vi "Open.vi"(8 "error in (no error)":errorcluster, 11 "reference in":refnum<class "GarageDoor.lvclass">) -> (0 "error out":errorcluster, 3 "reference out":refnum<class "GarageDoor.lvclass">)   [LabVIEW 2020, in "GarageDoor.lvclass"]
uses:
  GarageDoor.lvclass
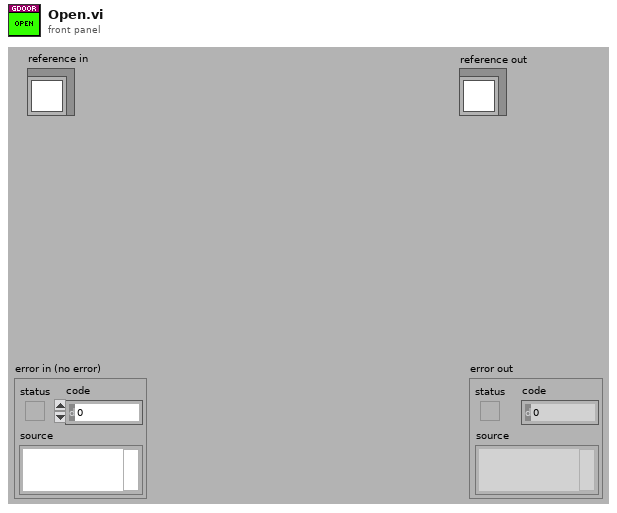
[diagram p1: front panel]
types:
  T1 = typedef "GarageDoor.lvclass/ObjectAttributes.ctl" = cluster{"None":bool}
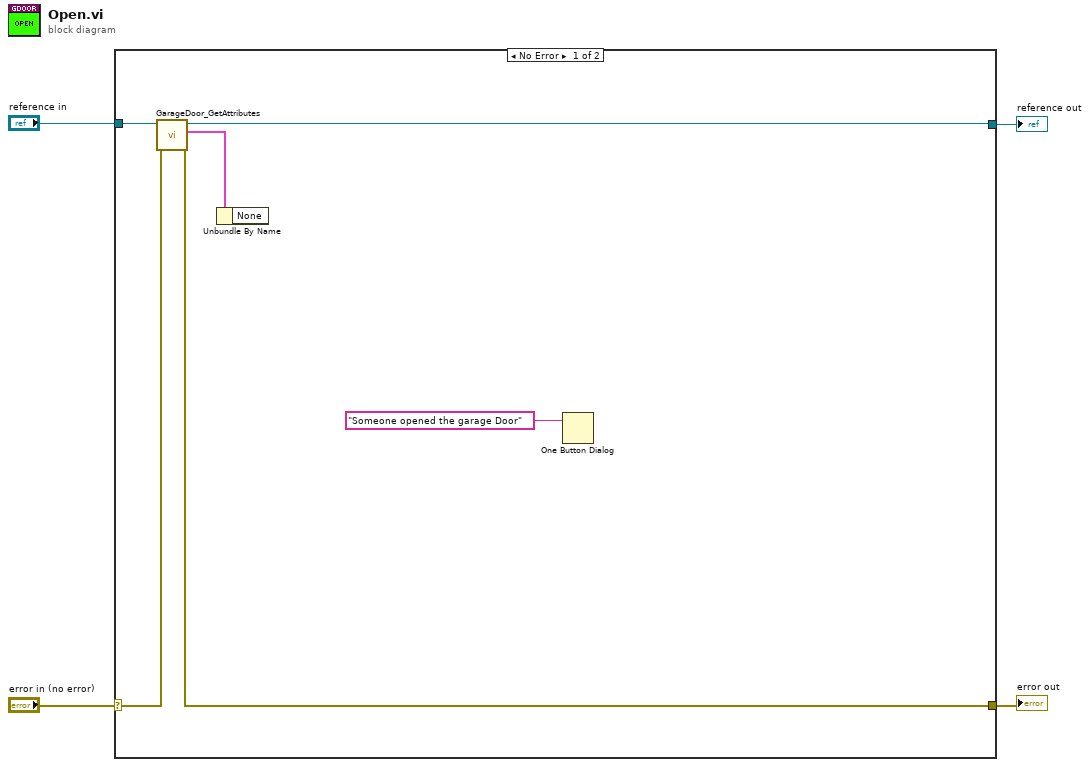
[diagram p0: block diagram]
diagram:
  n1 = case shown="No Error" "error in (no error)" {
    selector: "error in (no error)" -> [w9 w12]
    tunnel: [w6 w12] -> w3
    tunnel: [w7 w11] -> w1
    tunnel: "reference in" -> [w10 w11]
    frame No Error {
      n2 = call "GarageDoor_GetAttributes.vi"("error in (no error)"=w9, "reference in"=w10) -> ("error out"=w6:errorcluster, "Data"=w8:T1, "reference out"=w7:refnum<class "GarageDoor.lvclass">)  [unwired: 6 in, 1 out]
      n3 = Unbundle By Name(w8) -> ()  [unwired: 1 out]
      n4 = One Button Dialog(message="Someone opened the garage Door" ("TextIn")) -> ()  [unwired: 1 in, 1 out]
    }
    frame Error {
    }
  }
  "error out" <- w3
  "reference out" <- w1
